vi "AlliGator All ROIs Average Lifetimes.vi"(8 "error in (no error)":errorcluster, 10 "Lifetime Graph":refnum<vi>, 11 "AlliGator Internal Variables DVR":refnum<data-value>) -> (0 "error out":errorcluster, 1 "Message":string, 3 "AlliGator Internal Variables DVR":refnum<data-value>)   [LabVIEW 2021, in "AlliGator Decay Analysis.lvlib" / "AlliGator Decay Processing.lvlib"]
doc: "Computes an approximate average lifetime for all ROI decays, based on the integral under the curve and IRF information."
uses:
  AlliGator Decay Processing.lvlib
  AlliGator Internal Variables v2.ctl
  <vilib>/vision/Image Controls.llb/IMAQ Image.ctl
  AlliGator Gate Image Set.ctl
  AlliGator FLI Dataset Type.ctl
  AlliGator Data Series Type.ctl
  AlliGator Dataset Channel.ctl
  AlliGator Gate Arithmetic.ctl
  AlliGator Displayed Image.ctl
  Image/Named ROI Description.ctl
  AlliGator Decay Metadata v3.ctl
  AlliGator Decay Background Subtraction Info.ctl
  AlliGator Baseline Subtraction Method.ctl
  Graphs/XY Graph/XY Graph Plot Shift Parameters.ctl
  Graphs/XY Graph/XY Graph Plot Shift Method.ctl
  AlliGator Decay Extrapolation Parameters.ctl
  Phasor/Calibration Phasor (m, phi).ctl
  Phasor/Phasor Reference Series.ctl
  Phasor/Phasor Calibration Map v2.ctl
  Phasor/Phasor (g, s).ctl
  AlliGator Raw Phasor Plot Data v4.ctl
  Phasor/Phasor Standard Deviation Options.ctl
  AlliGator Phasor Multi-Harmonic Data.ctl
  Phasor/Phasor Harmonic Data.ctl
  AlliGator Decay Fit Options & Parameters v2.ctl
  Fits/IRF(X)PSED/Decay Fit Options v2.ctl
  Fits/Decay Convolution/Decay Model.ctl
  Fits/Residual Type.ctl
  Fits/IRF(X)PSED/Fit Weights Type.ctl
  Fits/Non-linear Fitting Method v2.ctl
  Fits/Fit Calculation Method.ctl
  Fits/Non-linear Fitting Algorithm.ctl
  AlliGator Decay Fit Parameter Constraints 2.ctl
  Fits/IRF(X)PSED/Decay Fit Parameters In List.ctl
  Fits/IRF(X)PSED/MLE Baseline Offset Type.ctl
  AlliGator Decay Preprocessing Parameters.ctl
  Fits/IRF(X)PSED/Decay Fit Parameters & Derived Quantities List.ctl
  AlliGator Variables List.ctl
  AlliGator Average Lifetime Options.ctl
  AlliGator Settings List.ctl
  Variant/Variant to Data/Variant to U16.vi
  Variant/Variant to Data/Variant to Boolean.vi
  AlliGator Abort.vi
  <vilib>/Utility/error.llb/Error Cluster From Error Code.vi
  <vilib>/ErrorRing/Error Ring.xnode
  AlliGator Globals, Variables & Constants.lvlib
  Image/Image.lvlib
  AlliGator Source Image.lvlib
  Strings/Strings.lvlib
  Time/Time.lvlib
  Graphs/XY Graph/XY Graph Add-Ons.lvlib
  AlliGator Settings.lvlib
  AlliGator Decay Preprocessing.lvlib
  Variant/Variant to Data/Variant to Data.lvlib
  Notebook/Notebook.lvlib
  Rich Text Box/Rich Text Box.lvlib
  Fits/Fits.lvlib
  AlliGator Decay Fit.lvlib
  AlliGator Decay Fit Parameter Map.lvlib
  Utilities/Utilities.lvlib
  GUI/GUI.lvlib
  Phasor/Phasor.lvlib
  AlliGator Files.lvlib
  AlliGator Internal Variables.lvlib
  AlliGator Phasor Graph.lvlib
  AlliGator Phasor Plot.lvlib
  AlliGator Dual-Channel Datasets.lvlib
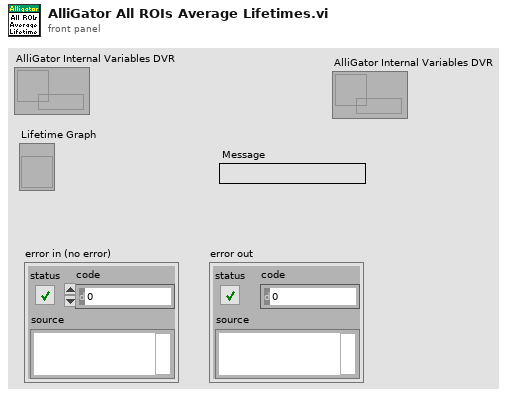
[diagram p1: front panel]
types:
  T1 = typedef "AlliGator Globals, Variables & Constants.lvlib/AlliGator Variables List.ctl" = enum16{"---- GUI ----", "Initialization Status", "State Indicators Refnum", "Original AlliGator Menu Items", "Current Action Loop State", "Script in progress", "Playback", "Loop Playback", "Search ROI Used", "Search ROI", "Decay Graph Max Legend Size", "Intensity Graph Max Legend Size", "Decay Statistics Graph Max Legend Size", "Phasor Graph Max Legend Size", "Phasor Ratio Graph Max Legend Size", "Lifetime Graph Max Legend Size", "---- Files ----", "Export Dataset Frames as Individual Files", "Show Batch Export Help Balloons", "Frames in Dataset", "ptu File Frame Start Indices", "Current Frame in Dataset", "Current Frame Timestamp", "------ Python Plugins ------", "Python Plugins Information", "Python Session", "Valid Python Session?", "---- Source Image ----", "Dataset Loaded", "Dataset Metadata", "Dataset Channel", "Dataset Data Description", "Background Dataset Metadata", "Background Dataset Channel", "Background Dataset Data Description", "Background File Subtraction", "Background File Path", "Background File Pile-up Correction", "Background File Pixel Well Capacity", "Background File Scaling Factor", "Source Image ROIs", "Current Source Image ROI", "Source Image ROI Event Refnum", "X_Source Image Display Range", "X_Source Image Palette Information", "Source Image Palette List", "Source Image Scale", "Current Dataset Load Settings", "Source Image:ROI Overlay Color", "---- Image Profile Window ----", "Image Profile:Overlay ROI in Source Image", "Image Profile Window Event Refnum", "Image Profile:IntensityType", "Image Profile:Intensity Average Type", "Image Profile:Intensity-weighted SDV", "Image Profile:Box Profile Type", "Image Profile Window Open", "Image Profile:Plotted Fit Parameter", "X_Type of Displayed Image", "X_Time Gate Slider", "Dataset Path", "Source Image Overlay to Erase", "Is Displayed Image Accumulated", "White Light Image Modified", "Mask Image Modified", "Macrotime Gate Separation", "------ Phasor Graph -------", "Phasor Graph:Show Line", "---- Phasor Plot ---", "Phasor Plot Parameters Changed", "FLI Dataset Modified since last Phasor Plot Calculation", "Phasor Harmonics Data", "Selected Phasor Harmonics", "Phasor Harmonic Manager Event Refnum", "Phasor Plot ROIs", "Current Phasor Plot ROI", "Phasor Plot ROI Event Refnum", "Phasor Plot Image Reference Points", "Phasor Plot Computed", "Phasor Plot Palette Information", "Phasor Plot Palette List", "Phasor Ratio Palette Information", "Phasor Ratio Palette List", "Phasor Image Scale", "Phasor Plot Image Overlay to Erase", "Phasor Plot Image Elements to Update", "Current Phasor Plot Calculation Parameters", "Current Phasor Calibration Options", "Reset Cumulated Phasor Plot", "Phasor Ratio Reference 1", "Phasor Ratio Lifetime Reference 1", "Phasor Ratio Reference 1 Frequency", "Phasor Ratio Reference 2", "Phasor Ratio Lifetime Reference 2", "Phasor Ratio Reference 2 Frequency", "---- Decay Analysis ----", "Number of Selected Decays to Fit", "LS Fit Results", "LAR Fit Results", "BS Fit Results", "Last Decay Max - Min", "Best Fit Parameters", "Best Fit Parameter Names", "Actual Size X", "Actual Size Y", "Binning X", "Binning Y", "Actual # Gates", "Dataset Number", "Gates to...", "Gates Skipped", "Gates to keep", "Gate Step", "Gate Separation", "Reversed Gates", "Pile-up Correction", "Pixel Well Capacity", "Background Subtracted", "Background Subtraction Method", "Background Definition Range", "Background File (deprecated)", "Number of Dataset Accumulated", "Array of Accumulated Dataset Paths", "Do Averaged Datasets", "Destination File Path", "Process Plot Target", "Use 1/D as Phasor Frequency", "---- Decay Fit Parameter Map -----", "Decay Fit Parameter Map Palette Information", "Decay Fit Parameter Map Palette List", "Local Decay Graph Window Event Refnum", "------- Local Decay Window ---------", "Use normalized IRF for convolution", "----- Miscellaneous ----", "Skippable Dialog Windows Status"}
  T2 = typedef "AlliGator Settings.lvlib/AlliGator Average Lifetime Options.ctl" = cluster{"Use Local IRF ":bool, "Use IRF Offset":bool, "Use Fixed Offset":bool, "Fixed Offset":dbl[unit], "Baseline %":dbl}
  T3 = typedef "AlliGator Settings.lvlib/AlliGator Settings List.ctl" = enum16{"GUI:Visible Settings Tab", "GUI:Last Run Version", "Source Image:Use Image Histogram for Contrast", "Source Image:Low Count Pixels Rejection Options", "Source Image:High Count Pixels Rejection Options", "Source Image:Use Image Brightness", "Source Image:Blend Overlay with Image Background", "Source Image:Use Fixed ROI Diameter", "Source Image:ROI Diameter", "Source Image:ROI Center Color", "Source Image:Peak Threshold", "Source Image:Intensity Threshold", "Source Image:Image Binning Options", "Source Image:Image Smoothing Options", "Source Image:Image Histogram Active", "Source Image:Invert Binary Mask", "Source Image:Hot Pixel Removal", "Source Image:Overlay Analyzed ROI Center", "Source Image:Auto-Adjust Contrast", "Source Image:Histogram Lower Percentile", "Source Image:Histogram Upper Percentile", "Source Image:Save Source Image", "Source Image:Scale Bar Options", "Source Image:Image Resolution (Pixel Size)", "Source Image:Flatfield Correction", "Source Image:Show Dead Left Columns Correction", "Source Image:Dead Left Columns Correction", "Source Image:Image Pre-Processing Operations Order", "Data Information:Gate Width", "Data Information:Nanotime Gate Separation", "Data Information:Macrotime Gate Separation", "Data Information:Gate Step", "Data Information:# Gates", "Data Information:Gate Image Exposure", "Data Information:Gate Image Integration", "Data Information:Gates to Skip", "Data Information:Gates to Keep", "Data Information:Define Gates to", "Data Information:Channel Name", "Data Information:Available Channel Names", "Data Information:Channel Arithmetic", "Data Information:Background File Subtraction", "Data Information:Background File", "Data Information:Background Scaling Factor", "Data Information:Background Pile-up Correction", "Data Information:Background Pixel Well Capacity", "Data Information:Laser Period", "Data Information:SYNC Period", "Data Information:Pile-up Correction", "Data Information:Pixel Well Capacity", "Data Information:Dataset Scaling Factor", "Fluorescence Decay_Decay Pre-Processing:Reverse Gates", "Fluorescence Decay_Decay Pre-Processing:Verbose Decay Pre-Processing", "Fluorescence Decay_Decay Pre-Processing:Use Decay Pre-Processing", "Fluorescence Decay_Decay Pre-Processing:Background Subtraction", "Fluorescence Decay_Decay Pre-Processing:Background Definition Range", "Fluorescence Decay_Decay Pre-Processing:Baseline Subtraction Method", "Fluorescence Decay_Decay Pre-Processing:Decay Pre-Processing Operations Order", "Fluorescence Decay_Decay Pre-Processing:Smoothing Parameter", "Fluorescence Decay_Decay Pre-Processing:Shift Decay", "Fluorescence Decay_Decay Pre-Processing:Decay Shift Parameters", "Fluorescence Decay_Decay Pre-Processing:Fold Decay", "Fluorescence Decay_Decay Pre-Processing:# Folds", "Fluorescence Decay_Decay Pre-Processing:1-Normalize Decay", "Fluorescence Decay_Decay Pre-Processing:[0-1]-Normalize Decay", "Fluorescence Decay_Decay Pre-Processing:Smoothen Decay", "Fluorescence Decay_Decay Pre-Processing:Extrapolate Decay", "Fluorescence Decay_Decay Pre-Processing:Use Periodicity", "Fluorescence Decay_Decay Pre-Processing:Use Cursors", "Fluorescence Decay_Decay Pre-Processing:Tail Fraction", "Fluorescence Decay_Decay Pre-Processing:Head Fraction", "Fluorescence Decay_Decay Pre-Processing:Additional Points", "Fluorescence Decay_Decay Pre-Processing:Straighten Decay", "Fluorescence Decay_Decay Pre-Processing:Constant Background", "Fluorescence Decay_Decay Pre-Processing:Pixel-Normalize Decay", "Fluorescence Decay_Advanced Analysis:Extract IRF instead of Decay", "Fluorescence Decay_Advanced Analysis:IRF Extraction Options", "Fluorescence Decay_Advanced Analysis:IRF Optimization Options", "Fluorescence Decay_Advanced Analysis:Square Pulse Options", "Fluorescence Decay_Advanced Analysis:IRF Order", "Fluorescence Decay_Advanced Analysis:IRF Time Constants", "Fluorescence Decay_Advanced Analysis:Wavelet Analysis Options", "Fluorescence Decay_Advanced Analysis:Average Lifetime Options", "Fluorescence Decay_Fit Options:Fit Options", "Fluorescence Decay_Fit Options:Use Legacy Fitting Approach", "Fluorescence Decay_Fit Options:Use Data Information Laser Period", "Fluorescence Decay_Fit Parameters:Displayed Fit Parameters", "Fluorescence Decay_Fit Parameters:Fit Parameter Constraints", "Fluorescence Decay_Fit Parameters:Export Tabulated Results", "Fluorescence Decay_Fit Parameters:MLE Baseline Offset Type", "Fluorescence Decay_Fit Parameters:MLE Baseline Offset", "Fluorescence Decay_Fit Parameters:Guess Parameter Names", "Fluorescence Decay_Fit Parameters:Guess Parameter Values", "Fluorescence Decay_Fit Parameters:Guess Parameters Options", "Fluorescence Decay_Styles:Show Last Decay Only", "Fluorescence Decay_Styles:Decay Graph Color Array", "Fluorescence Decay:Decay Graph Active", "Fluorescence Decay Statistics:Min Peak Value", "Fluorescence Decay Statistics:Reject Low Decay Peak Pixels", "Fluorescence Decay Statistics:Reject High Decay Peak Pixels", "Fluorescence Decay Statistics:Max Peak Value", "Time Traces:Use File Timestamp", "Time Traces:Time Step", "Time Traces:Use Intensity Correction File", "Time Traces:Intensity Correction File", "Phasor Plot:Phasor Plot Smoothing Options", "Phasor Plot:Phasor Plot Size", "Phasor Plot:Phasor Plot Graphics Options", "Phasor Plot:Cumulative Phasor Plot", "Phasor Plot:Use Phasor Brightness", "Phasor Plot:Blend Overlay with Phasor Background", "Phasor Plot:Save Phasor Plot", "Phasor Plot:Show References", "Phasor Plot:Phasor Ratio Decay Range", "Phasor Plot:Exponential Fading", "Phasor Plot:Phasor Ratio Reference Colors", "Phasor Plot:Reference Radius", "Phasor Plot:Show Color Map Vertices", "Phasor Plot:Phasor Plot Active", "Phasor Plot:Phasor Ratio Color Map Type", "Phasor Plot:Phasor Ratio Color Map", "Phasor Plot:Phasor Ratio Display Range", "Phasor Plot:Selected Image ROI(s)", "Phasor Plot:All Image ROIs", "Phasor Plot:Selected Phasor Plot ROI(s)", "Phasor Plot:All Phasor Plot ROIs", "Phasor Plot:Phasor Ratio Color-Coded Quantity", "Phasor Plot:Store Phasor Harmonics", "Phasor Plot:Draw Reference Segment", "Phasor Plot:User-Defined Quantity", "Phasor Graph:Phasor Frequency", "Phasor Graph:Phasor Ratio Type", "Phasor Graph:Pixel-level Phasor Computation", "Phasor Graph:Save Phasor Graph", "Phasor Graph:Phasor Graph Active", "Phasor Graph:Phasor SDV Options", "Phasor Calibration:Use Backup Calibration if needed", "Phasor Graph:Define Shortest Lifetime as", "Phasor Calibration:Backup Calibration Type", "Phasor Calibration:Calibration Type", "Phasor Calibration:Calibration Lifetime", "Phasor Calibration:Calibration Map Algorithm", "Single-Exponential Phasor Locus (SEPL):Gate Parameters", "Single-Exponential Phasor Locus (SEPL):User-defined Gate", "Single-Exponential Phasor Locus (SEPL):User-defined IRF", "Single-Exponential Phasor Locus (SEPL):Phasor Parameters", "Single-Exponential Phasor Locus (SEPL):Decay & IRF Parameters", "Single-Exponential Phasor Locus (SEPL):Display Parameters", "Lifetime Analysis:Decay Analysis Parameters", "Lifetime Analysis:Lifetime Map Active", "Plugins:Python Settings", "Miscellaneous:Verbose Mode", "Miscellaneous:Beep after Script", "Miscellaneous:Saved Image File Format", "Miscellaneous:Exported Gate Image Settings", "Miscellaneous:Include Loading in Timing", "Miscellaneous:Verbose Settings Mode", "Miscellaneous:Histogram Options", "Miscellaneous:Beep on Error", "Miscellaneous:# Logical Processors Used", "Miscellaneous:ROI Description Max Characters", "Miscellaneous:Verbose Error Mode", "Miscellaneous:Transparent Mask Color"}
  T4 = typedef "IMAQ Image.ctl" = refnum<image>
  T5 = typedef "Image.lvlib/Named ROI Description.ctl" = cluster{"ROI Descriptor":T6, "ROI Name":string, "Overlay Color":u32}
  T6 = typedef "ROI Descriptor" = cluster{"Global Rectangle":i32[], "Contours":cluster{"ID":enum32{"External", "Internal"}, "Type":u32, "Coordinates":i32[]}[]}
  T7 = typedef "Fits.lvlib/Decay Model.ctl" = enum16{"1-Exponential", "2-Exponentials"}
  T8 = typedef "AlliGator Decay Fit Parameter Map.lvlib/AlliGator Decay Fit Options & Parameters v2.ctl" = cluster{"SYNC Period":dbl[unit], "Fit Options":T9, "Fit Parameter Constraints":T15[], "MLE Baseline Offset":dbl, "MLE Baseline Offset Type":T17}
  T9 = typedef "Fits.lvlib/Decay Fit Options v2.ctl" = cluster{"Show Fit Residuals":bool, "Fit Model":T7, "Residual Type":T10, "Max Decay Percentile":dbl, "Min Decay Percentile":dbl, "Show Full Decay":bool, "Weights":T11, "Fitting Method":T12, "Compute Parameter Uncertainties":bool, "Periodic Boundaries":bool, "Model Calculation":T13, "Period":dbl[unit], "Termination Criteria":cluster{"Max Iterations":i32, "Max Function Calls":i32, "Max Time":dbl[unit], "Function Tolerance":dbl, "Parameter Tolerance":dbl, "Gradient Tolerance":dbl, "Min Lambda":dbl, "Max Lambda":dbl, "Initial Tick Count":u32}, "Offset Resolution":dbl[unit], "Use Local IRF":bool, "Fitting Algorithm":T14}
  T10 = typedef "Fits.lvlib/Residual Type.ctl" = enum16{"Standard", "Normalized", "Reduced"}
  T11 = typedef "Fits.lvlib/Fit Weights Type.ctl" = enum16{"Unweighted", "1/Variance", "Best of All"}
  T12 = typedef "Fits.lvlib/Non-linear Fitting Method v2.ctl" = enum16{"Least Square", "Least Absolute Residual", "Bisquare", "MLE", "-", "Best of All"}
  T13 = typedef "Fits.lvlib/Fit Calculation Method.ctl" = enum16{"Simulation", "Convolution", "Integration"}
  T14 = typedef "Fits.lvlib/Non-linear Fitting Algorithm.ctl" = enum16{"Levenberg-Marquardt", "Trust-Region Dogleg"}
  T15 = typedef "AlliGator Decay Analysis.lvlib/AlliGator Decay Fit.lvlib/AlliGator Decay Fit Parameter Constraints 2.ctl" = cluster{"Fit Parameter":T16, "Min Value":dbl, "Max Value":dbl, "Global":bool, "Used":bool}
  T16 = typedef "Fits.lvlib/Decay Fit Parameters In List.ctl" = enum16{"Offset", "Baseline", "A_1", "tau_1", "A_2", "tau_2"}
  T17 = typedef "Fits.lvlib/MLE Baseline Offset Type.ctl" = enum32{"Absolute", "Percentage"}
  T18 = typedef "AlliGator Internal Variables.lvlib/AlliGator Internal Variables v2.ctl" = cluster{"Displayed Image":T4, "White Light Image":T4, "Mask Image":T4, "ROI Mask Image":T4, "Current Dataset Images 1":T19, "Background Dataset Images 1":T19, "Current Dataset Images 2":T19, "Background Dataset Images 2":T19, "Current Dataset Arithmetic Images":T19, "Accumulated Dataset Images 1":T19, "Accumulated Dataset Images 2":T19, "Accumulated Dataset Arithmetic Images":T19, "Phasor Plot Image":T4, "Decay Fit Parameter Map Image":T4, "Single Data Point Path":path, "White Light Image Path":path, "Mask Image Path":path, "Time-Series Folder":path, "[Time-Series Paths]":path[], "Current Dataset":i32, "Single Dataset Type":T20, "Current Folder":string, "AlliGator Data Series Type":T21, "# Datasets":i32, "Dual-Channel Dataset":bool, "Selected Channel Name":string, "Dataset Channel":T22, "Channel Arithmetic":T23, "Dual-Channel Background Dataset":bool, "Background Channel":T22, "Dual-Channel Accumulated Dataset":bool, "Start Time":dbl, "[Time-Series Timestamps]":dbl[], "[Intensity Corrections]":dbl[], "Time Series Script":bool, "Type of Displayed Image":T24, "Gate Image Slide":u16, "# Gates":i32, "ROIs":T5[], "ROI Decay":cluster{"t Array":dbl[], "I Array":dbl[]}, "Valid Decay":bool, "Decay  Metadata":T25, "Reference Decay Plot Name":string, "Reference Decay":cluster{"t Array":dbl[], "I Array":dbl[]}, "Decay Shift Plot":cluster{"Time Stamps":dbl[], "Decay Shifts":dbl[]}, "[Decays Max Values]":sgl[], "[Decays Min Values]":sgl[], "Calibration Phasor":T31, "Calibration Phasor Series":T32, "Phasor Calibration Map":T33, "Calibration Map MD5 Digest":string, "Last Raw Phasor":T34, "Last Calibrated Phasor":T34, "Last Calibrated Phasor SDV":T34, "Phasor Graph:Phasor Plot":cluster{"g Array":dbl[], "s Array":dbl[]}, "Phasor Graph:Phasor SDV Plot":cluster{"g Array":dbl[], "s Array":dbl[]}, "[Phasor Graph:Raw Phasor Plots]":T35[], "Phasor Plot locked to Ref 1":i32, "[Phasor Plot(s) locked to Ref 1]":i32[], "[Phasor Plot(s) locked to Ref 2]":i32[], "[Pixel Phasors]":T34[], "[[Sum Image]]":dbl[][], "[[CSG Phasors]]":csg[][], "[[Valid Pixel?]]":bool[][], "I/m/phi Dataset":cluster{"I/m/phi Dataset?":bool, "Base Frequency":dbl[unit], "Harmonic Orders":u8[]}, "Multi Phasor Plot Data":T37, "Decay Fit Options & Parameters":T8, "Fit Options: Decay Preprocessing Parameters":T39, "Fit Options: Reference Decay":cluster{"t Array":dbl[], "I Array":dbl[]}, "Is Full Image Parameters Map":bool, "Is Single-Pixels Parameters Map":bool, "NLSF Parameters Map X Resolution":i32, "NLSF Parameters Map Y Resolution":i32, "[Single Decay Fit Parameters]":dbl[], "Fit Model":T7, "[[Multiple Decays Fit Parameters]]":dbl[][], "[[Multiple Decays Fit Parameter SDVs]]":dbl[][], "[[IRFs]]":dbl[][], "IRF Array Time Axis":dbl[], "Decay Array Time Axis":dbl[], "[Decay Fit Parameter Names]":T40[], "[[Phasor Ratios]]":dbl[][], "[[Average Lifetimes]]":dbl[][], "Amplitude Weighted Average Lifetime":bool, "[Decay Sum]":dbl[], "[[User-defined Quantities]]":dbl[][], "User-defined Quantity":string}
  T19 = typedef "AlliGator Internal Variables.lvlib/AlliGator Gate Image Set.ctl" = cluster{"SGL Image Max":T4, "SGL Image Sum":T4, "SGL Gate Images":T4[], "SGL Image Min":T4}
  T20 = typedef "AlliGator Files.lvlib/AlliGator FLI Dataset Type.ctl" = enum16{"HDF5 FLI Dataset", "Gate Image Folder", ".sdt FLI Dataset (Becker & Hickl)", ".ptu FLI Dataset (PicoQuant)", "SS1 FLI Dataset", "SS2 FLI Dataset", "I/m/phi Dataset", ".bin FLI Dataset (PicoQuant Binned)", ".bin FLI Dataset (Piccolo Binned)"}
  T21 = typedef "AlliGator Files.lvlib/AlliGator Data Series Type.ctl" = enum16{"Not a Supported Series", "Gate Images Folder Series", "SwissSPAD 2 Dataset Series", "B&H FLI Dataset Series", "PicoQuant PTU FLI Dataset Series", "PicoQuant BIN FLI Dataset Series", "Piccolo hist BIN FLI Dataset Series", "HDF5 FLI Dataset Series"}
  T22 = typedef "AlliGator Dual-Channel Datasets.lvlib/AlliGator Dataset Channel.ctl" = enum16{"G2", "INT"}
  T23 = typedef "AlliGator Settings.lvlib/AlliGator Gate Arithmetic.ctl" = enum16{"None", "INT-G2", "G2/INT*<INT>", "(1 - G2/INT)*<INT>"}
  T24 = typedef "AlliGator Source Image.lvlib/AlliGator Displayed Image.ctl" = enum16{"Single Gate", "Sum of All Gates", "Max of All Gates", "Min of All Gates", "-", "White Ligth Image", "Mask Image"}
  T25 = typedef "AlliGator Phasor Graph.lvlib/AlliGator Decay Metadata v3.ctl" = cluster{"ROI Descriptor":T6, "ROI Center":cluster{"X":i32, "Y":i32}, "Decay Background Subtraction Info":T26, "Decay Reverted":bool, "Decay Smoothened":bool, "Decay Straightened":bool, "Fitted Tau (Decay Straightening)":dbl, "Decay Shift Parameters":T28, "Decay Shifted":bool, "Decay Extrapolated":bool, "Decay Extrapolation Parameters":T30, "Decay Normalized":bool, "Fold Decay":bool, "# Folds":u32}
  T26 = typedef "AlliGator Decay Analysis.lvlib/AlliGator Decay Preprocessing.lvlib/AlliGator Decay Background Subtraction Info.ctl" = cluster{"Laser Period":dbl[unit], "Gate Duration":dbl[unit], "Baseline Subtraction Method":T27, "Background Definition Range":cluster{"Min Gate":dbl[unit], "Max Gate":dbl[unit]}, "Total Intensity w/o Bkgd Subtraction":dbl, "Bkgd-subtracted Intensity (exp)":dbl, "# Data Points":i32, "Background/Gate":dbl, "Fitted Lifetime":dbl[unit], "Bkgd-subtracted Intensity (theo)":dbl}
  T27 = typedef "AlliGator Decay Analysis.lvlib/AlliGator Decay Preprocessing.lvlib/AlliGator Baseline Subtraction Method.ctl" = enum16{"Mean", "Min", "Square Gated Single-Exponential", "File", "Constant"}
  T28 = typedef "XY Graph Add-Ons.lvlib/XY Graph Plot Shift Parameters.ctl" = cluster{"Type":T29, "Shift":dbl[unit], "Threshold":dbl, "Rotate":bool}
  T29 = typedef "XY Graph Add-Ons.lvlib/XY Graph Plot Shift Method.ctl" = enum16{"Default", "CFD", "Threshold", "Cross-Correlation"}
  T30 = typedef "AlliGator Decay Analysis.lvlib/AlliGator Decay Preprocessing.lvlib/AlliGator Decay Extrapolation Parameters.ctl" = cluster{"Additional Points":u32, "Head Fraction":dbl, "Fitted Tau":dbl, "Use Periodicity":bool, "Use Cursors":bool, "Tail Fraction":dbl}
  T31 = typedef "Phasor.lvlib/Calibration Phasor (m, phi).ctl" = cluster{"m":dbl, "phi":dbl, "Phasor Frequency":dbl[unit], "Reference Lifetime":dbl[unit]}
  T32 = typedef "Phasor.lvlib/Phasor Reference Series.ctl" = cluster{"m Array":dbl[], "phi Array":dbl[], "Phasor Frequency":dbl[unit], "Calibration Lifetime":dbl[unit]}
  T33 = typedef "Phasor.lvlib/Phasor Calibration Map v2.ctl" = cluster{"Phasor Frequency":dbl[unit], "Calibration Lifetime":dbl[unit], "ROI Centers":cluster{"X":i32, "Y":i32}[], "ROI Descriptors":T6[], "Map Resolution X":i32, "Map Resolution Y":i32, "z Array":cdb[]}
  T34 = typedef "Phasor.lvlib/Phasor (g, s).ctl" = cluster{"g":dbl, "s":dbl}
  T35 = typedef "AlliGator Phasor Graph.lvlib/AlliGator Raw Phasor Plot Data v4.ctl" = cluster{"Phasor Plot Name":string, "Raw Phasor Plot":T34[], "Phasor Frequency":dbl[unit], "[Decay Metadata]":T25[], "Raw Phasor Plot SDV":T34[], "Phasor SDV Options":T36, "[Calibration Phasor]":T31[]}
  T36 = typedef "Phasor.lvlib/Phasor Standard Deviation Options.ctl" = cluster{"Compute Estimated SDV":bool, "# Replicas":u32, "Use Estimated Average Phasor":bool}
  T37 = typedef "AlliGator Phasor Plot.lvlib/AlliGator Phasor Multi-Harmonic Data.ctl" = cluster{"Base Frequency":dbl[unit], "# Harmonics":u8, "Harmonic Orders":u8[], "Phasor Plot Settings Checksum":u64, "Phasor Harmonic Data Array":T38[]}
  T38 = typedef "Phasor.lvlib/Phasor Harmonic Data.ctl" = cluster{"Phasor Harmonic Name":string, "Phasor Plot Settings Checksum":u64, "Phasor Frequency":dbl[unit], "Base Frequency":dbl[unit], "Harmonic Order":u8, "Phasor Plot Parameters":string, "Phasor Array [[CSG]]":csg[][], "Dataset File Path":path}
  T39 = typedef "AlliGator Decay Analysis.lvlib/AlliGator Decay Preprocessing.lvlib/AlliGator Decay Preprocessing Parameters.ctl" = cluster{"Background Subtraction":bool, "Straighten Decay":bool, "Reverse Gates":bool, "1-Normalized Decay":bool, "Smoothen Decay":bool, "Smoothing Parameter":dbl, "Shift Decay":bool, "Decay Shift Parameters":T28, "Extrapolate Decay":bool, "Additional Points":u32, "Head Fraction":dbl, "Pixel-Normalize Decay":bool, "Use Periodicity":bool, "Use Cursors":bool, "Tail Fraction":dbl, "Use Decay Pre-Processing":bool, "Fold Decay":bool, "# Folds":u32, "[0-1]-Normalized Decay":bool}
  T40 = typedef "Fits.lvlib/Decay Fit Parameters & Derived Quantities List.ctl" = enum16{"Offset", "Baseline", "A_1", "tau_1", "A_2", "tau_2", "<tau>_a", "f1_a", "f2_a", "<tau>_i", "f1_i", "f2_i", "-", "R^2", "Chi^2"}
  T41 = typedef "AlliGator Settings.lvlib/AlliGator Pixel Counts Constraints.ctl" = cluster{"High Count Pixels Rejection Options":T42, "Low Count Pixels Rejection Options":T43}
  T42 = typedef "AlliGator Settings.lvlib/AlliGator High Count Pixels Rejection Options.ctl" = cluster{"Background High Threshold Factor":dbl, "Fixed High Background Threshold":dbl, "Reject High Count Pixels":bool, "High Percentile":dbl}
  T43 = typedef "AlliGator Settings.lvlib/AlliGator Low Count Pixels Rejection Options.ctl" = cluster{"Background Low Threshold Factor":dbl, "Fixed Low Background Threshold":dbl, "Reject Low Count Pixels":bool, "Low Percentile":dbl}
  T44 = cluster{"Decay Peak Constraint":bool, "Min":dbl, "Max":dbl}
  T45 = typedef "Rich Text Box.lvlib/Text Formatting.ctl" = cluster{"Font":string, "Text Color":T46, "Text Background Color":T46, "Text Style":enum16{"Regular", "Bold", "Italic", "Underline", "Strikeout"}, "Font Size (Points)":dbl, "Text Alignment":i32}
  T46 = typedef "Rich Text Box.lvlib/Text Colors.ctl" = enum16{"Unchanged", "Black", "Blue", "Brown", "Gray", "Green", "Orange", "Pink", "Red", "White"}
  T47 = typedef "XY Graph Add-Ons.lvlib/XY Graph Refnum.ctl" = refnum<vi>
  T48 = cluster{"t Axis":dbl[], "ROI Intensity Array":dbl[]}
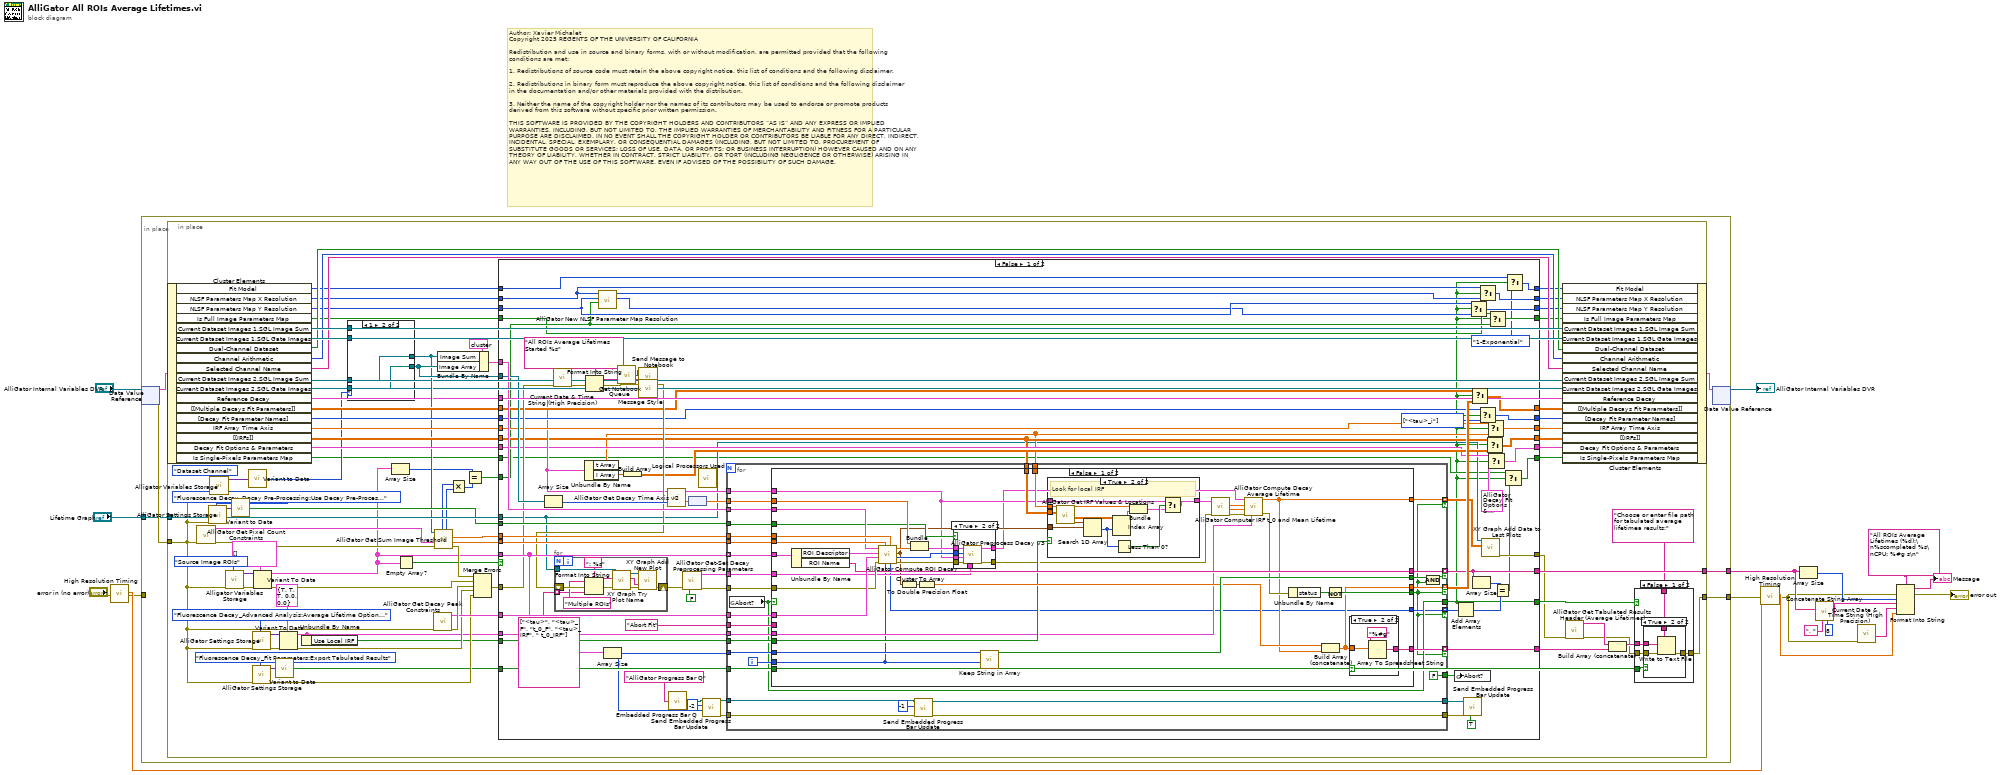
[diagram p0: block diagram]
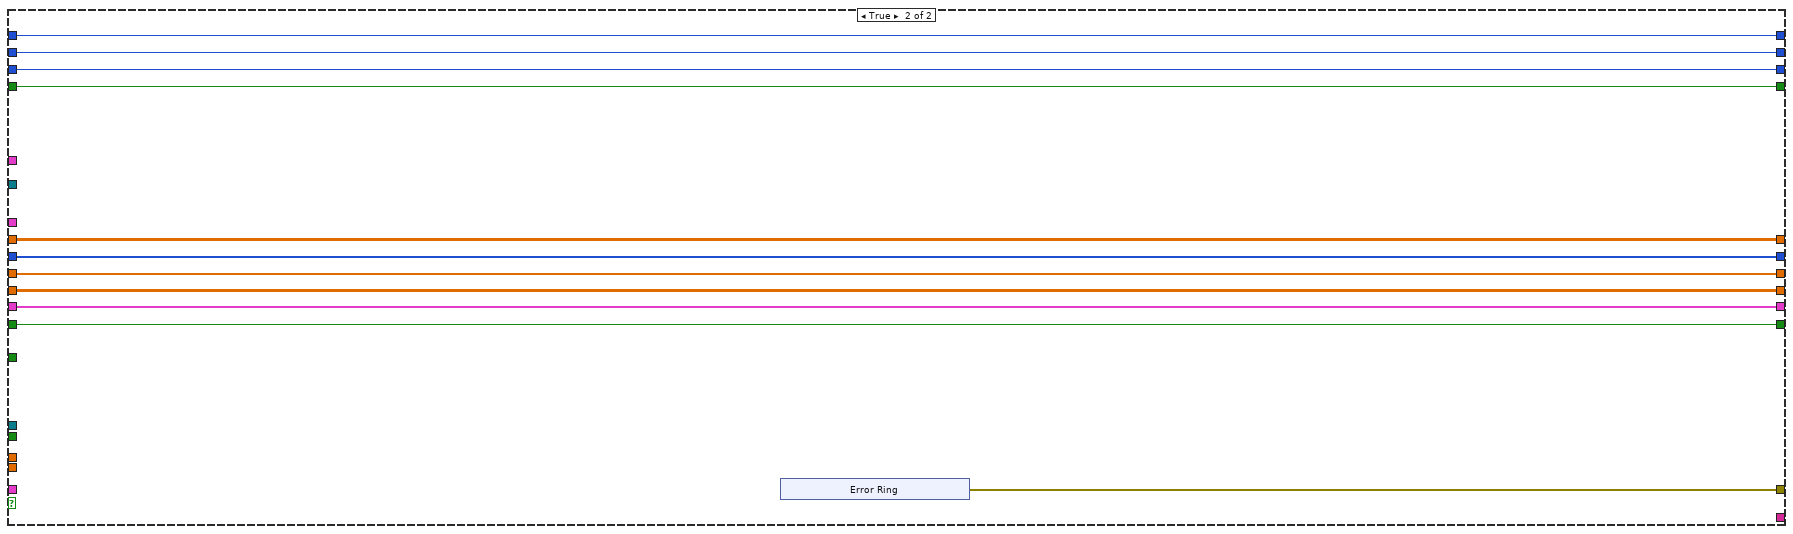
[diagram p7: hidden frame]
diagram:
  # "Author: Xavier Michalet\nCopyright 2025 REGENTS OF THE UNIVERSITY OF CALIFORNIA\n\nRedistribution and use in source and binary forms, with or without modification, are permitted provided that the following conditions are met:\n\n1. Redistributions of source code must retain the above copyright notice, this list of conditions and the following disclaimer.\n\n2. Redistributions in binary form must reproduce the above copyright notice, this list of conditions and the following disclaimer in the documentation and/or other materials provided with the distribution.\n\n3. Neither the name of the copyright holder nor the names of its contributors may be used to endorse or promote products derived from this software without specific prior written permission.\n\nTHIS SOFTWARE IS PROVIDED BY THE COPYRIGHT HOLDERS AND CONTRIBUTORS “AS IS” AND ANY EXPRESS OR IMPLIED WARRANTIES, INCLUDING, BUT NOT LIMITED TO, THE IMPLIED WARRANTIES OF MERCHANTABILITY AND FITNESS FOR A PARTICULAR PURPOSE ARE DISCLAIMED. IN NO EVENT SHALL THE COPYRIGHT HOLDER OR CONTRIBUTORS BE LIABLE FOR ANY DIRECT, INDIRECT, INCIDENTAL, SPECIAL, EXEMPLARY, OR CONSEQUENTIAL DAMAGES (INCLUDING, BUT NOT LIMITED TO, PROCUREMENT OF SUBSTITUTE GOODS OR SERVICES; LOSS OF USE, DATA, OR PROFITS; OR BUSINESS INTERRUPTION) HOWEVER CAUSED AND ON ANY THEORY OF LIABILITY, WHETHER IN CONTRACT, STRICT LIABILITY, OR TORT (INCLUDING NEGLIGENCE OR OTHERWISE) ARISING IN ANY WAY OUT OF THE USE OF THIS SOFTWARE, EVEN IF ADVISED OF THE POSSIBILITY OF SUCH DAMAGE."
  n1 = call "High Resolution Timing.vi"("Error In"="error in (no error)") -> ("elapsed (relative) seconds"=w12:dbl, "Error Out"=w7:errorcluster)  [unwired: 16 in, 1 out]
  n2 = in-place {
    in-place-border: [w22] -> w5
    in-place-border: [w21] -> w9
    in-place-border: w7 -> [_]
    in-place-border: "Lifetime Graph" -> [w19]
    n3 = in-place-dvr #1("AlliGator Internal Variables DVR") -> (w24:T18, w20:errorcluster)
    n4 = in-place {
      in-place-border: w20 -> [w41]
      in-place-border: [w81] -> w22
      in-place-border: [w92] -> w21
      in-place-border: w19 -> [w89]
      n5 = in-place-cluster #2(w24) -> ("Fit Model"=w26:T7, "NLSF Parameters Map X Resolution"=w32:i32, "NLSF Parameters Map Y Resolution"=w31:i32, "Is Full Image Parameters Map"=w40:bool, "Current Dataset Images 1.SGL Image Sum"=w61:T4, "Current Dataset Images 1.SGL Gate Images"=w60:T4[], "Dual-Channel Dataset"=w56:bool, "Channel Arithmetic"=w55:T23, "Selected Channel Name"=w54:string, "Current Dataset Images 2.SGL Image Sum"=w59:T4, "Current Dataset Images 2.SGL Gate Images"=w58:T4[], "Reference Decay"=w47:cluster{"t Array":dbl[], "I Array":dbl[]}, "[[Multiple Decays Fit Parameters]]"=w74:dbl[][], "[Decay Fit Parameter Names]"=w71:T40[], "IRF Array Time Axis"=w69:dbl[], "[[IRFs]]"=w68:dbl[][], "Decay Fit Options & Parameters"=w65:T8, "Is Single-Pixels Parameters Map"=w27:bool)
      n6 = call "AlliGator Get Pixel Count Constraints.vi"("error in (no error)"=w41) -> ("error out"=w99:errorcluster, "Pixel Count Constraints"=w100:T41)  [unwired: 9 in]
      n7 = call "AlliGator Settings Storage.vi"("AlliGator Settings List"=AlliGator_Settings_List."Fluorescence Decay_Decay Pre-Processing:Use Decay Pre-Processing", "Error In"=w41) -> ("Variant Data out"=w77:variant)  [unwired: 8 in, 1 out]
      n8 = call "Alligator Variables Storage.vi"("AlliGator Variable"=AlliGator_Variables_List."Dataset Channel" ("Alligator Variable"), "Error In"=w41) -> ("Data out"=w43:variant)  [unwired: 7 in, 2 out]
      n9 = call "Alligator Variables Storage.vi"("AlliGator Variable"=AlliGator_Variables_List."Source Image ROIs" ("Alligator Variable"), "Error In"=w41) -> ("Error Out"=w102:errorcluster, "Data out"=w103:variant)  [unwired: 7 in, 1 out]
      n10 = call-poly "Variant to Data.vi"("Variant"=w77) -> ("Value"=w75:bool)  [unwired: 8 in]
      n11 = call-poly "Variant to Data.vi"("Variant"=w43) -> ("U16 Value"=w42:u16)  [unwired: 8 in]
      n12 = call "AlliGator Settings Storage.vi"("AlliGator Settings List"=AlliGator_Settings_List."Fluorescence Decay_Advanced Analysis:Average Lifetime Options", "Error In"=w41) -> ("Error Out"=w53:errorcluster, "Variant Data out"=w50:variant)  [unwired: 8 in]
      n13 = call "AlliGator Settings Storage.vi"("AlliGator Settings List"=AlliGator_Settings_List."Fluorescence Decay_Fit Parameters:Export Tabulated Results", "Error In"=w41) -> ("Error Out"=w86:errorcluster, "Variant Data out"=w87:variant)  [unwired: 8 in]
      n14 = Variant To Data(error in=w102, type=T5[] [] ("Stored ROIs in"), Variant=w103) -> (data=w36:T5[], error out=w98:errorcluster)
      n15 = call-poly "Variant to Data.vi"("Variant"=w87) -> ("Value"=w79:bool)  [unwired: 8 in]
      n16 = Variant To Data(error in=w53, type=T2 {"Use Local IRF "=TRUE, "Use IRF Offset"=TRUE, "Use Fixed Offset"=TRUE, "Fixed Offset"=0.0, "Baseline %"=0.0} ("Average Lifetime Options"), Variant=w50) -> (data=w48:T2, error out=w51:errorcluster)
      n17 = Unbundle By Name(w48) -> ("Use Local IRF"=w46:bool)
      n18 = case shown="1" w42 {
        tunnel: [w106 w108] -> w62
        tunnel: w61 -> [w106 _]
        tunnel: [w105 w107] -> w63
        tunnel: w60 -> [w105 _]
        tunnel: w59 -> [_ w108]
        tunnel: w58 -> [_ w107]
        frame 0, Default {
        }
        frame 1 {
        }
      }
      n19 = Array Size(array=w36) -> (size(s)=w35:i32)
      n20 = Empty Array?(array=w36) -> (empty?=w45:bool)
      n21 = call "AlliGator Get Decay Peak Constraints.vi"("error in (no error)"=w41) -> ("Error Out"=w95:errorcluster, "Decay Peak Constraints"=w94:T44)  [unwired: 9 in]
      n22 = call "AlliGator Get Sum Image Threshold.vi"("error in (no error)"=w99, "Pixel Counts Constraints"=w100, "Image in"=w62) -> ("error out"=w91:errorcluster, "Pixel Threshold Low"=w96:sgl, "Pixel Threshold High"=w97:sgl, "Y Resolution"=w38:i32, "X Resolution"=w37:i32)  [unwired: 2 in, 2 out]
      n23 = Bundle By Name(cluster=cluster{"Image Sum":T4, "Image Array":T4[]} {"Image Sum"=refnum, "Image Array"=[]} ("Images"), "Image Sum"=w62, "Image Array"=w63) -> (w93:cluster{"Image Sum":T4, "Image Array":T4[]})
      n24 = Multiply(x=w37, y=w38) -> (x*y=w34:i32)
      n25 = Equal?(x=w35, y=w34) -> (x = y?=w33:bool)
      n26 = Merge Errors(w91, w98, w95, w51, w86) -> (w90:errorcluster)
      n27 = case shown="False" w45 {
        tunnel: w97 -> [w187 _]
        tunnel: w96 -> [w186 _]
        tunnel: w94 -> [w185 _]
        tunnel: w93 -> [w184 _]
        tunnel: w63 -> [w183 _]
        tunnel: w47 -> [w157 _]
        tunnel: [w116 _] -> w92
        tunnel: w90 -> [w166 _]
        tunnel: w89 -> [w141 _]
        tunnel: [w178 _] -> w85
        tunnel: [w112 _] -> w82
        tunnel: [w140 w305] -> w73
        tunnel: w79 -> [w177 _]
        tunnel: [w164 w306] -> w78
        tunnel: w36 -> [w176 _]
        tunnel: w75 -> [w175 _]
        tunnel: w74 -> [w163 w306]
        tunnel: w71 -> [w162 w304]
        tunnel: [w161 w304] -> w70
        tunnel: w69 -> [w160 w303]
        tunnel: w68 -> [w148 w302]
        tunnel: [w159 w303] -> w67
        tunnel: [w158 w302] -> w66
        tunnel: w65 -> [w154 w301]
        tunnel: [w153 w301] -> w64
        tunnel: w48 -> [w146 _]
        tunnel: w46 -> [w145 _]
        tunnel: w40 -> [w120 w300]
        tunnel: [w128 w300] -> w39
        tunnel: w33 -> [w121 _]
        tunnel: w32 -> [w125 w299]
        tunnel: w31 -> [w123 w298]
        tunnel: [w127 w299] -> w30
        tunnel: [w126 w298] -> w29
        tunnel: [w119 w297] -> w28
        tunnel: w27 -> [w118 w297]
        tunnel: w26 -> [w111 w296]
        tunnel: [w110 w296] -> w25
        frame False {
          w149 = T40[] [enum."<tau>_i"] items=["Offset", "Baseline", "A_1", "tau_1", "A_2", "tau_2", "<tau>_a", "f1_a", "f2_a", "<tau>_i", "f1_i", "f2_i", "-", "R^2", "Chi^2"] ("f")
          n28 = Array Size(array=w183) -> (size(s)=w182:i32)
          n29 = call "Current Date & Time String (High Precision).vi"("Error In"=w166) -> ("Error Out"=w170:errorcluster, "on <Date> at <Time>"=w150:string)  [unwired: 7 in, 2 out]
          n30 = Unbundle By Name(w157) -> ("t Array"=w147:dbl[], "I Array"=w156:dbl[])
          n31 = Format Into String(format string="All ROIs Average Lifetimes Started %s", error in=w170, w150) -> (resulting string=w171:string, error out=w169:errorcluster)  [unwired: 1 in]
          n32 = call "AlliGator New NLSF Parameter Map Resolution.vi"("Is Full Image Parameter Map"=w121, "Old NLSF Parameters Map Y Resolution"=w123, "Old NLSF Parameters Map X Resolution"=w125) -> (2:"New NLSF Parameters Map X Resolution"=w122:i32, 3:"New NLSF Parameters Map X Resolution"=w124:i32)  [unwired: 7 in]
          n33 = Array Size(array=w176) -> (size(s)=w134:i32)
          n34 = call "Get Notebook Queue.vi"() -> ("Notebook Queue"=w168:refnum<queue>)  [unwired: 9 in]
          n35 = Build Array(w156) -> (w155:dbl[][])
          n36 = call "Message Style.vi"() -> ("Message Formatting"=w173:T45)
          n37 = call "Send Message to Notebook.vi"("Text Formatting"=w173, "Error In"=w169, "Message"=w171, "Notebook Queue"=w168) -> ("Error Out"=w167:errorcluster)  [unwired: 4 in, 1 out]
          n38 = for {
            tunnel: w141 -> [w195]
            shift-right: [w197] -> w174
            shift-left: w167 -> [w193]
            tunnel: string[] ["<tau>", "<tau>_F", "t_0_F", "<tau>_IRF", " t_0_IRF"] ("initial string") -> [w188] mode=indexing
            n39 = Format Into String(format string=": %s", initial string="Multiple ROIs", error in=w193, w188) -> (resulting string=w191:string, error out=w192:errorcluster)
            n40 = call "XY Graph Try Plot Name.vi"("Error In"=w192, "Plot Name in"=w191, "XY Graph Refnum"=w195) -> ("Error Out"=w196:errorcluster, "Plot Name out"=w198:string, "XY Graph Refnum"=w189:T47)  [unwired: 5 in, 1 out]
            n41 = call "XY Graph Add New Plot.vi"("Multiplot XY Graph"=w189, "New Plot Name in"=w198, "error in (no error)"=w196) -> ("error out"=w197:errorcluster)  [unwired: 9 in, 3 out]
          }
          n42 = call "AlliGator Get Decay Time Axis v2.vi"("Number of Gates"=w182) -> ("t Array"=w181:dbl[unit][])  [unwired: 14 in]
          n43 = call "Embedded Progress Bar Q.vi"("Progress Bar Queue Name"="AlliGator Progress Bar Q") -> ("Progress Bar Queue"=w137:refnum<queue>)  [unwired: 6 in]
          n44 = call "AlliGator Get-Set Decay Preprocessing Parameters.vi"("Get (F)/Set"=FALSE, "Error In"=w174) -> ("Error Out"=w138:errorcluster, "Decay Preprocessing Parameters out"=w152:T39)  [unwired: 8 in]
          n45 = node(w181) -> (w180:dbl[])
          n46 = call "Logical Processors Used.vi"() -> ()  [unwired: 6 in, 1 out]
          n47 = call "Send Embedded Progress Bar Update.vi"("Max Iterations N"=w134, "Current Iteration i (i or -1: standard or || iteration; 0 or -2: first standard or || iteration)"=-2 ("Current Iteration i (i or -1: standard or || iteration; 0 or -2: first standard or || iteration)"), "Progress Bar Queue in"=w137) -> ("Error Out"=w132:errorcluster, "Progress Bar Queue out"=w133:refnum<queue>)  [unwired: 7 in]
          n48 = for {
            tunnel: w176 -> [w231] mode=indexing
            tunnel: w187 -> [w230]
            tunnel: w186 -> [w229]
            tunnel: w184 -> [w228]
            tunnel: w185 -> [w227]
            tunnel: w180 -> [w225]
            tunnel: w157 -> [w211]
            tunnel: [w224] -> w116 mode=indexing if=w217
            tunnel: w138 -> [w226]
            tunnel: [FALSE ("Abort?")] -> w179
            tunnel: "Abort Fit" ("Abort Button Name (Abort)") -> [w222]
            tunnel: [w221] -> w178 mode=indexing if=w199
            tunnel: w177 -> [w220]
            tunnel: [w207] -> w112
            tunnel: [w208] -> w165 mode=indexing if=w199
            tunnel: w134 -> [w219]
            tunnel: w175 -> [w215]
            tunnel: w152 -> [w214]
            tunnel: w148 -> [w213]
            tunnel: w147 -> [w212]
            tunnel: w146 -> [w209]
            tunnel: w145 -> [w210]
            tunnel: [w206] -> w142 mode=indexing if=w199
            tunnel: w133 -> [w204]
            tunnel: w132 -> [w203]
            tunnel: [w202] -> w130
            tunnel: [w201] -> w129
            tunnel: [w200] -> w117 mode=indexing if=w199
            i -> [w218]
            n49 = global read "AlliGator Abort.vi" "Abort?"() -> (w207:bool)
            n50 = case shown="False" w207 {
              tunnel: w231 -> [w271 _]
              tunnel: w230 -> [w270 _]
              tunnel: w229 -> [w269 _]
              tunnel: w228 -> [w268 _]
              tunnel: w227 -> [w267 _]
              tunnel: w226 -> [w266 _]
              tunnel: w225 -> [w263 _]
              tunnel: [w259 _] -> w224
              tunnel: w222 -> [_ _]
              tunnel: [w258 _] -> w221
              tunnel: w220 -> [w257 _]
              tunnel: w219 -> [w256 _]
              tunnel: w218 -> [w232 _]
              tunnel: [w255 _] -> w216
              tunnel: [w254 _] -> w199
              tunnel: w215 -> [w251 _]
              tunnel: w214 -> [w250 _]
              tunnel: w213 -> [w248 _]
              tunnel: w212 -> [w247 _]
              tunnel: w211 -> [w246 _]
              tunnel: w210 -> [w241 _]
              tunnel: w209 -> [w240 _]
              tunnel: [w236 _] -> w208
              tunnel: [w235 _] -> w206
              tunnel: [w233 _] -> w200
              frame False {
                n51 = Unbundle By Name(w271) -> ("ROI Descriptor"=w265:T6, "ROI Name"=w259:string)
                n52 = call "AlliGator Compute ROI Decay.vi"("Pixel Threshold High"=w270, "Loop ID"=w232, "Pixel Threshold Low"=w269, "error in (no error)"=w266, "Decay Peak  Constraints"=w267, "ROI Descriptor"=w265, "Images"=w268) -> ("error out"=w264:errorcluster, "# Valid Pixels"=w260:i32, "ROI Center"=w249:cluster{"X":i32, "Y":i32}, "Decay Points"=w262:dbl[], "# Pixels"=w233:i32)
                n53 = Cluster To Array(cluster=w249) -> (array=w253:i32[])
                n54 = Bundle(w263, "Decay Points"=w262) -> (w261:cluster{dbl[], "Decay Points":dbl[]})  [unwired: 1 in]
                n55 = To Double Precision Float(number=w253) -> (double precision float=w252:dbl[])
                n56 = case shown="True" w251 {
                  tunnel: w264 -> [w284 w292]
                  tunnel: w261 -> [w285 w291]
                  tunnel: w260 -> [_ w290]
                  tunnel: [w284 w289] -> w234
                  tunnel: w246 -> [_ w288]
                  tunnel: [w285 w287] -> w239
                  tunnel: w250 -> [_ w286]
                  frame False {
                  }
                  frame True {
                    n57 = call "AlliGator Preprocess Decay v3.vi"("Decay Preprocessing Parameters"=w286, "Error In"=w292, "Time-Gated Reference Decay"=w288, "# Pixels"=w290, "Decay (in)"=w291) -> ("Error Out"=w289:errorcluster, "Decay (out)"=w287:T48)  [unwired: 3 in, 2 out]
                  }
                }
                n58 = call "Keep String in Array.vi"("Current Index"=w232, "Number of Elements"=w256) -> ("Keep String"=w255:bool)  [unwired: 9 in]
                n59 = case shown="True" w241 {
                  tunnel: w248 -> [_ w283]
                  tunnel: w246 -> [w272 w278]
                  tunnel: [w272 w277] -> w245
                  tunnel: w247 -> [_ w276]
                  tunnel: w249 -> [_ w273]
                  frame False {
                  }
                  frame True {
                    # "Look for local IRF"
                    n60 = call "AlliGator Get IRF Values & Locations.vi"("[IRF Data]"=w283) -> ("IRF Locations"=w282:cluster{"X":i32, "Y":i32}[], "[IRF Values]"=w281:dbl[][])  [unwired: 9 in]
                    n61 = Search 1D Array(1D array=w282, element=w273) -> (index of element=w280:i32)  [unwired: 1 in]
                    n62 = Index Array(array=w281, index (row)=w280) -> (element=w275:dbl[])  [unwired: 1 in]
                    n63 = Less Than 0?(x=w280) -> (x < 0?=w279:bool)
                    n64 = Bundle("t Array"=w276, "[IRF Values]"=w275) -> (w274:cluster{"t Array":dbl[], "[IRF Values]":dbl[]})  [unwired: 1 in]
                    n65 = Select(t=w278, s=w279, f=w274) -> (s? t:f=w277:cluster{"t Array":dbl[], "[IRF Values]":dbl[]})
                  }
                }
                n66 = call "AlliGator Computer IRF t_0 and Mean Lifetime.vi"("error in"=w234, "Reference Decay"=w245) -> ("error out"=w242:errorcluster, "t_0"=w243:dbl, "<tau>_IRF"=w244:dbl)  [unwired: 7 in]
                n67 = call "AlliGator Compute Decay Average Lifetime.vi"("Average Lifetime Options"=w240, "error in (no error)"=w242, "t_0_IRF"=w243, "<tau>_IRF"=w244, "Plot"=w239) -> ("error out"=w238:errorcluster, "Average Lifetime Outputs"=w235:dbl[])  [unwired: 5 in]
                n68 = Unbundle By Name(w238) -> ("status"=w237:bool)
                n69 = Build Array (concatenate)(w252, w235) -> (w236:dbl[])
                n70 = Not(x=w237) -> (.not. x?=w254:bool)
                n71 = case shown="True" w257 {
                  tunnel: [_ w295] -> w258
                  tunnel: w236 -> [_ w294]
                  frame False {
                  }
                  frame True {
                    n72 = Array To Spreadsheet String(array=w294, 3:"%#g" ("format string")) -> (spreadsheet string=w295:string)  [unwired: 1 in]
                  }
                }
              }
              frame True {
              }
            }
            n73 = call "Send Embedded Progress Bar Update.vi"("Error In"=w203, "Current Iteration i (i or -1: standard or || iteration; 0 or -2: first standard or || iteration)"=-1 ("Current Iteration i (-1: || iteration, -2: first || iteration)"), "Progress Bar Queue in"=w204) -> ("Error Out"=w201:errorcluster, "Progress Bar Queue out"=w202:refnum<queue>)  [unwired: 7 in]
            n74 = Compound Arithmetic op=AND(w216, w199) -> (w217:bool)
          }
          n75 = global write "AlliGator Abort.vi" "Abort?"(w179) -> ()
          n76 = Add Array Elements(numeric array=w117) -> (sum=w114:i32)
          n77 = call "Send Embedded Progress Bar Update.vi"("Stop Progress Bar (F)"=TRUE, "Error In"=w129, "Progress Bar Queue in"=w130) -> ()  [unwired: 7 in, 2 out]
          n78 = Select(t=w123, s=w112, f=w122) -> (s? t:f=w126:i32)
          n79 = Select(t=w163, s=w112, f=w165) -> (s? t:f=w164:dbl[][])
          n80 = Array Size(array=w116) -> (size(s)=w115:i32)
          n81 = Select(t=w162, s=w112, f=w149) -> (s? t:f=w161:T40[])
          n82 = Select(t=w125, s=w112, f=w124) -> (s? t:f=w127:i32)
          n83 = call "XY Graph Add Data to Last Plots.vi"("Plots Data Array"=w142, "XYGraph in"=w141) -> ("error out"=w140:errorcluster)  [unwired: 9 in]
          n84 = Select(t=w148, s=w112, f=w155) -> (s? t:f=w158:dbl[][])
          n85 = Select(t=w160, s=w112, f=w147) -> (s? t:f=w159:dbl[])
          n86 = Select(t=w154, s=w112, f=T8 {"SYNC Period"=0.0, "Fit Options"={"Show Fit Residuals"=FALSE, "Fit Model"=enum."1-Exponential", "Residual Type"=enum."Standard", "Max Decay Percentile"=0.0, "Min Decay Percentile"=0.0, "Show Full Decay"=FALSE, "Weights"=enum."Unweighted", "Fitting Method"=enum."Least Square", "Compute Parameter Uncertainties"=FALSE, "Periodic Boundaries"=FALSE, "Model Calculation"=enum."Simulation", "Period"=0.0, "Termination Criteria"={"Max Iterations"=0, "Max Function Calls"=0, "Max Time"=0.0, "Function Tolerance"=0.0, "Parameter Tolerance"=0.0, "Gradient Tolerance"=0.0, "Min Lambda"=0.0, "Max Lambda"=0.0, "Initial Tick Count"=0}, "Offset Resolution"=0.0, "Use Local IRF"=FALSE, "Fitting Algorithm"=enum."Levenberg-Marquardt"}, "Fit Parameter Constraints"=[], "MLE Baseline Offset"=0.0, "MLE Baseline Offset Type"=enum."Absolute"}) -> (s? t:f=w153:T8)
          n87 = Select(t=w120, s=w112, f=w121) -> (s? t:f=w128:bool)
          n88 = Equal?(x=w115, y=w114) -> (x = y?=w113:bool)
          n89 = Select(t=w118, s=w112, f=w113) -> (s? t:f=w119:bool)
          n90 = Select(t=w111, s=w112, f=Decay_Model."1-Exponential") -> (s? t:f=w110:T7)
        }
        frame True {
          n91 = xnode "Error Ring"() -> ("error out"=w305:errorcluster)
        }
      }
      n92 = in-place-cluster #2("Fit Model"=w25, "NLSF Parameters Map X Resolution"=w30, "NLSF Parameters Map Y Resolution"=w29, "Is Full Image Parameters Map"=w39, "Current Dataset Images 1.SGL Image Sum"=w61, "Current Dataset Images 1.SGL Gate Images"=w60, "Dual-Channel Dataset"=w56, "Channel Arithmetic"=w55, "Selected Channel Name"=w54, "Current Dataset Images 2.SGL Image Sum"=w59, "Current Dataset Images 2.SGL Gate Images"=w58, "Reference Decay"=w47, "[[Multiple Decays Fit Parameters]]"=w78, "[Decay Fit Parameter Names]"=w70, "IRF Array Time Axis"=w67, "[[IRFs]]"=w66, "Decay Fit Options & Parameters"=w64, "Is Single-Pixels Parameters Map"=w28) -> (w23:T18)
      n93 = call "AlliGator Get Tabulated Results Header (Average Lifetimes).vi"("Error In"=w73) -> ("Error Out"=w72:errorcluster, "Tabulated Results Header"=w84:string)  [unwired: 9 in]
      n94 = Build Array (concatenate)(w84, w85) -> (w83:string[])
      n95 = case shown="False" w82 {
        tunnel: w83 -> [w315 _]
        tunnel: [w314 w321] -> w81
        tunnel: w72 -> [w313 w321]
        tunnel: "Choose or enter file path for tabulated average lifetimea results:" ("prompt (Choose or enter file path)") -> [w312 _]
        tunnel: w79 -> [w311 _]
        frame False {
          n96 = case shown="True" w311 {
            tunnel: w315 -> [_ w320]
            tunnel: [w316 w319] -> w314
            tunnel: w313 -> [w316 w318]
            tunnel: w312 -> [_ w317]
            frame False {
            }
            frame True {
              n97 = Write to Text File(prompt (Choose or enter file path)=w317, text=w320, error in=w318) -> (error out=w319:errorcluster)  [unwired: 1 in, 2 out]
            }
          }
        }
        frame True {
        }
      }
    }
    n98 = in-place-dvr #1(w23) -> (→"AlliGator Internal Variables DVR":refnum<data-value>)  [unwired: 1 out]
  }
  n99 = call "High Resolution Timing.vi"("relative seconds (NaN)"=w12, "Error In"=w5) -> ("elapsed (relative) seconds"=w11:dbl, "Error Out"=w6:errorcluster)  [unwired: 15 in, 1 out]
  n100 = Array Size(array=w9) -> (size(s)=w8:i32)
  n101 = call "Concatenate String Array.vi"("Max Number of Elements (None: -1)"=8 ("Max Number of Elements (None: 1)"), "Separator (TAB)"=", ", "String Array"=w9) -> ("Formatted String"=w10:string)  [unwired: 8 in]
  n102 = call "Current Date & Time String (High Precision).vi"("Error In"=w6) -> ("on <Date> at <Time>"=w1:string)  [unwired: 7 in, 3 out]
  n103 = Format Into String(format string="All ROIs Average Lifetimes (%d):\n%scompleted %s\nCPU: %#g s\n", error in=w6, w8, w10, w1, w11) -> (resulting string=→"Message":string, error out=→"error out":errorcluster)  [unwired: 1 in]
